vi "Init AutoComplete.vi"(8 "error in (no error)":errorcluster, 11 "Editor in":refnum<class "Editor.lvclass">) -> (0 "error out":errorcluster, 3 "Editor out":refnum<class "Editor.lvclass">)   [LabVIEW 2020, in "VolatusGUIEditor.lvlib" / "Editor.lvclass"]
uses:
  Editor.lvclass
  Editor.lvclass/Editor.ctl
  lv-autocomplete/AutoComplete/Shared Options/Shared Options.lvclass
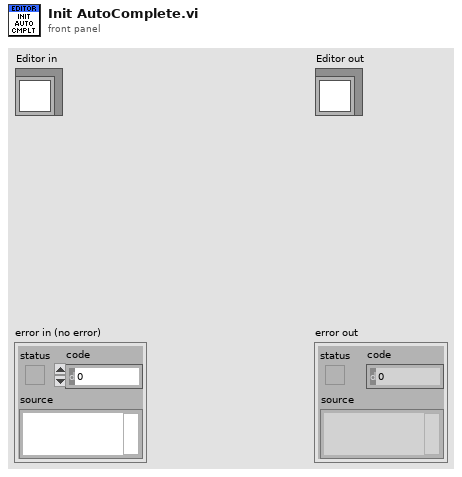
[diagram p1: front panel]
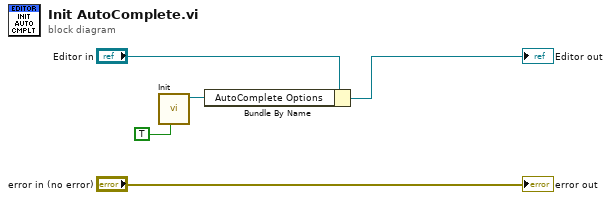
[diagram p0: block diagram]
diagram:
  n1 = call "Init.vi"("Allow Undefined Values (F)"=TRUE) -> ("Shared Config out"=w2:refnum<class "Shared Options.lvclass">)  [unwired: 9 in, 1 out]
  n2 = Bundle By Name(cluster="Editor in", "AutoComplete Options"=w2) -> (→"Editor out":refnum<class "Editor.lvclass">)
  "error out" <- "error in (no error)"
